vi "Get Status From String.vi"(10 "Status type":refnum<class "Status.lvclass">, 11 "data string":string) -> (2 "Status String":string, 3 "Item Name":string)   [LabVIEW 2017, in "Message Interface.lvlib" / "Status.lvclass"]
uses:
  Status.lvclass
  C:/Users/Public/Documents/wc/BuildFarm/src/LabVIEW/vi.lib/BenjaminR/Build Farm/Classes/Message Interface/iMessage/iMessage.lvclass
  Status.lvclass/Status.ctl
  iMessage/iMessage.lvclass
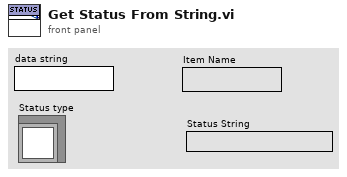
[diagram p1: front panel]
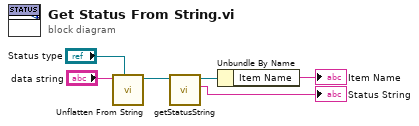
[diagram p0: block diagram]
diagram:
  n1 = call "Unflatten From String.vi"("iMessage in"="Status type", "binary string"="data string") -> ("iMessage out"=w3:refnum<class "Status.lvclass">)  [unwired: 8 in, 1 out]
  n2 = call-dynamic "getStatusString.vi"("Status in"=w3) -> ("Status String"=→"Status String":string, "Status out"=w2:refnum<class "Status.lvclass">)  [unwired: 8 in, 1 out]
  n3 = Unbundle By Name(w2) -> ("Item Name"=→"Item Name":string)
